vi "get sensor location.vi"(9 "reading":T1, 12 "magnetometer x locations":dbl[](array[numeric])=[0.0, -22.5, -22.5, 45.0], 13 "magnetometer y locations":dbl[](array[numeric])=[0.0, 38.971, -38.971, 0.0], 14 "magnetometer z locations":dbl[](array[numeric])=[0.0, 38.971, -38.971, 0.0]) -> (10 "location":cluster{"x":dbl, "y":dbl, "z":dbl})   [LabVIEW 2017]
uses:
  typedefs/reading.ctl
  typedefs/readingType.ctl
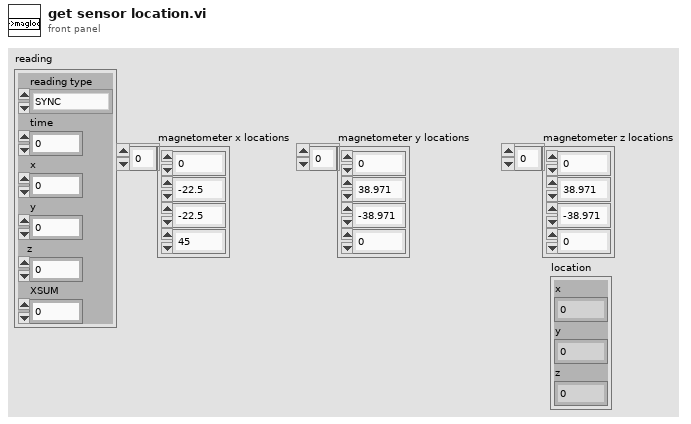
[diagram p1: front panel]
types:
  T1 = typedef "reading.ctl" = cluster{"reading type":T2, "time":fxp<+,48,48>, "x":sgl, "y":sgl, "z":sgl, "XSUM":u8}
  T2 = typedef "readingType.ctl" = enum8{"SYNC", "DETVAL", "COILI", "MAGVEC", "ACCVEC", "CROSSING", "MAGVEC0", "MAGVEC1", "MAGVEC2", "MAGVEC3", "MAGVEC4", "MAGVEC5", "MAGVEC6", "MAGVEC7"}
  T3 = cluster{"Numeric":dbl, "Numeric":dbl, "Numeric":dbl}
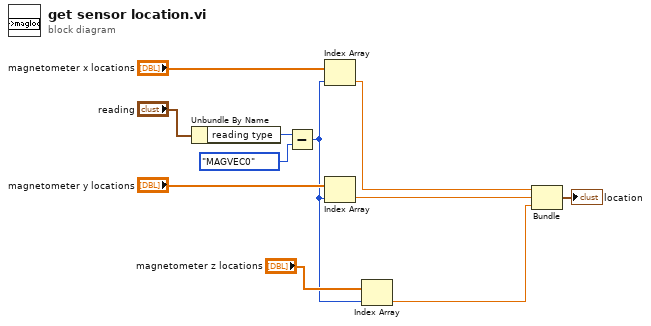
[diagram p0: block diagram]
diagram:
  n1 = Unbundle By Name("reading") -> ("reading type"=w10:T2)
  n2 = Subtract(x=w10, y=readingType."MAGVEC0") -> (x-y=w5:u8)
  n3 = Index Array(array="magnetometer x locations", index=w5) -> (element=w4:dbl)
  n4 = Index Array(array="magnetometer y locations", index=w5) -> (element=w3:dbl)
  n5 = Index Array(array="magnetometer z locations", index=w5) -> (element=w2:dbl)
  n6 = Bundle("Numeric"=w4, "Numeric"=w3, "Numeric"=w2) -> (→"location":T3)  [unwired: 1 in]
